vi "test1-SystemLevelModuleInListModuleAPI.vi"(8 "error in (no error)":errorcluster, 11 "TestCase in":refnum<class "testcase-CSMSystemLevelModule.lvclass">) -> (0 "error out":errorcluster, 3 "TestCase out":refnum<class "testcase-CSMSystemLevelModule.lvclass">)   [LabVIEW 2017, in "testcase-CSMSystemLevelModule.lvclass"]
uses:
  testcase-CSMSystemLevelModule.lvclass
  src/user.lib/_NEVSTOP/Communicable State Machine(CSM)/_Support/Typedef/_CSM_List Module Scope.ctl
  <vilib>/addons/_JKI Toolkits/VI Tester/TestCase.llb/TestCase.lvclass
  src/user.lib/_NEVSTOP/Communicable State Machine(CSM)/Communicable State Machine.lvlib
  C:/Program Files (x86)/National Instruments/LabVIEW 2017/vi.lib/addons/_JKI Toolkits/VI Tester/TestCase.llb/TestCase.lvclass
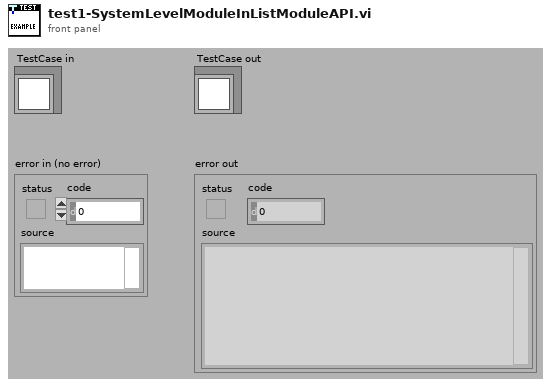
[diagram p1: front panel]
types:
  T1 = typedef "Communicable State Machine.lvlib/_CSM_List Module Scope.ctl" = enum16{"Normal", "System Only", "All"}
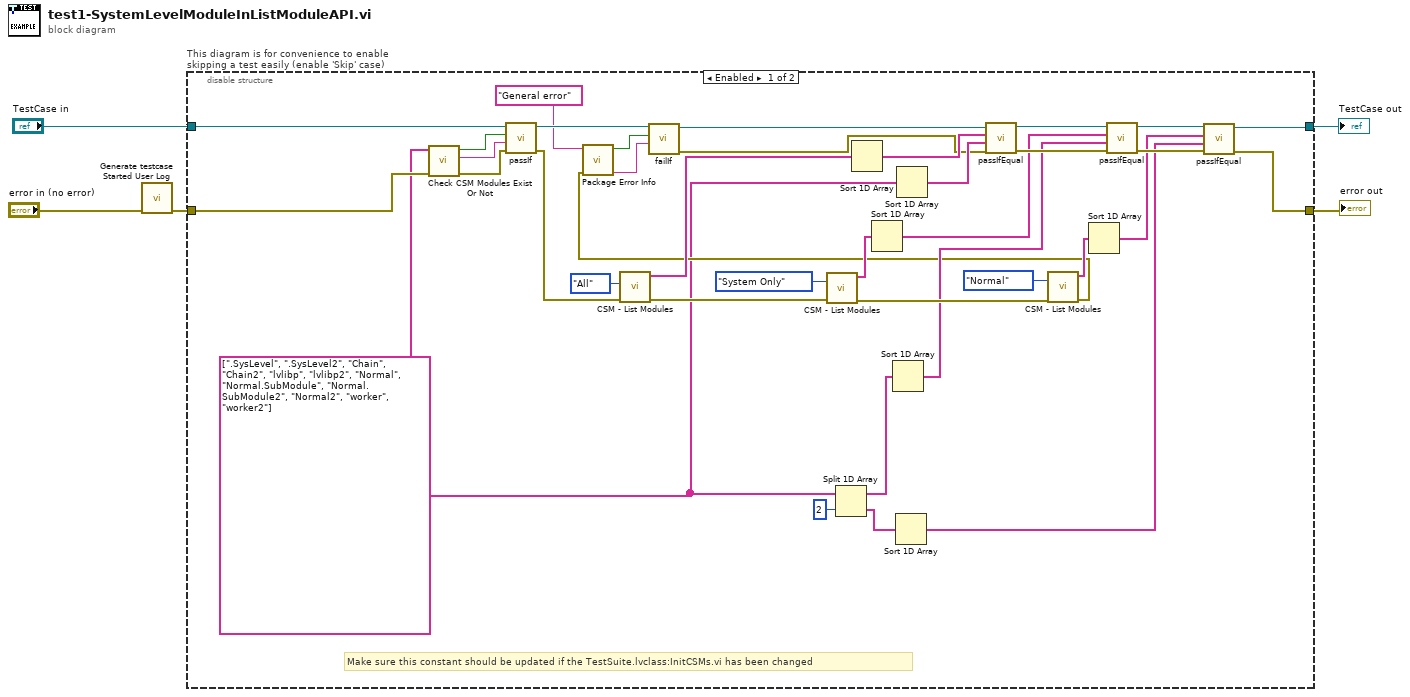
[diagram p0: block diagram]
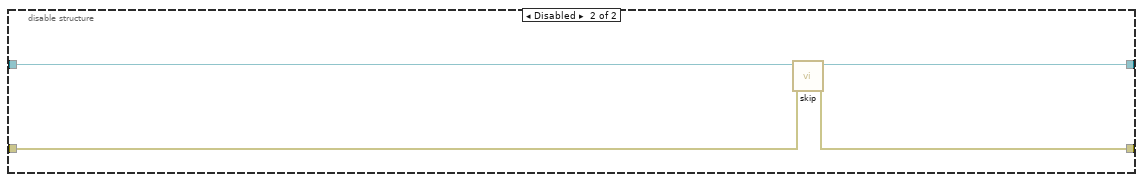
[diagram p2: hidden frame]
diagram:
  n1 = call "Generate testcase Started User Log.vi"("Error In"="error in (no error)") -> ("error out"=w1:errorcluster)  [unwired: 10 in]
  n2 = disable-structure "This diagram is for convenience to enable skipping a test easily (enable 'Skip' case)" shown="Enabled" {
    disable-tunnel: "TestCase in" -> [w16 w46]
    disable-tunnel: [w32 w44] -> w2
    disable-tunnel: [w29 w45] -> w4
    disable-tunnel: w1 -> [w15 w43]
    frame Enabled {
      w6 = string[] [".SysLevel", ".SysLevel2", "Chain", "Chain2", "lvlibp", "lvlibp2", "Normal", "Normal.SubModule", "Normal.SubModule2", "Normal2", "worker", "worker2"] ("Module Names in All Scope")
      # "Make sure this constant should be updated if the TestSuite.lvclass:InitCSMs.vi has been changed"
      n3 = call "Check CSM Modules Exist Or Not.vi"("error in"=w15, "CSM names in"=w6) -> ("error out"=w17:errorcluster, "Debug string"=w18:string, "All Modules Exist?"=w19:bool)  [unwired: 7 in]
      n4 = call-dynamic "passIf.vi"("error in (no error)"=w17, "message (\"\")"=w18, "pass"=w19, "TestCase in"=w16) -> ("error out"=w14:errorcluster, "TestCase out"=w11:refnum<class "testcase-CSMSystemLevelModule.lvclass">)  [unwired: 6 in]
      n5 = call "CSM - List Modules.vi"("Error In"=w14, "Scope (Normal)"=_CSM_List_Module_Scope."All") -> ("error out"=w39:errorcluster, "Module Names"=w37:string[])  [unwired: 8 in]
      n6 = call "CSM - List Modules.vi"("Error In"=w39, "Scope (Normal)"=_CSM_List_Module_Scope."System Only") -> ("error out"=w38:errorcluster, "Module Names"=w28:string[])  [unwired: 8 in]
      n7 = Split 1D Array(array=w6, index=2) -> (first subarray=w24:string[], second subarray=w23:string[])
      n8 = Sort 1D Array(array=w37) -> (sorted array=w36:string[])
      n9 = Sort 1D Array(array=w28) -> (sorted array=w27:string[])
      n10 = Sort 1D Array(array=w24) -> (sorted array=w26:string[])
      n11 = Sort 1D Array(array=w23) -> (sorted array=w20:string[])
      n12 = Sort 1D Array(array=w6) -> (sorted array=w35:string[])
      n13 = call "CSM - List Modules.vi"("Error In"=w38, "Scope (Normal)"=_CSM_List_Module_Scope."Normal") -> ("error out"=w9:errorcluster, "Module Names"=w22:string[])  [unwired: 8 in]
      n14 = call "Package Error Info.vi"("error in"=w9, "String in"="General error") -> ("packed error info out"=w12:string, "error status"=w13:bool)  [unwired: 8 in]
      n15 = call-dynamic "failIf.vi"("message (\"\")"=w12, "fail"=w13, "TestCase in"=w11) -> ("error out"=w7:errorcluster, "TestCase out"=w10:refnum<class "testcase-CSMSystemLevelModule.lvclass">)  [unwired: 7 in]
      n16 = call-dynamic "passIfEqual.vi"("error in (no error)"=w7, "y"=w35, "x"=w36, "TestCase in"=w10) -> ("error out"=w31:errorcluster, "TestCase out"=w34:refnum<class "testcase-CSMSystemLevelModule.lvclass">)  [unwired: 6 in]
      n17 = Sort 1D Array(array=w22) -> (sorted array=w21:string[])
      n18 = call-dynamic "passIfEqual.vi"("error in (no error)"=w31, "y"=w26, "x"=w27, "TestCase in"=w34) -> ("error out"=w30:errorcluster, "TestCase out"=w33:refnum<class "testcase-CSMSystemLevelModule.lvclass">)  [unwired: 6 in]
      n19 = call-dynamic "passIfEqual.vi"("error in (no error)"=w30, "y"=w20, "x"=w21, "TestCase in"=w33) -> ("error out"=w29:errorcluster, "TestCase out"=w32:refnum<class "testcase-CSMSystemLevelModule.lvclass">)  [unwired: 6 in]
    }
    frame Disabled {
      # "skip test result while test is under development"
      n20 = call <vilib>:"skip.vi"("error in (no error)"=w43, "TestCase in"=w46) -> ("error out"=w45:errorcluster, "TestCase out"=w44:refnum<class "testcase-CSMSystemLevelModule.lvclass">)  [unwired: 8 in]
    }
  }
  "error out" <- w4
  "TestCase out" <- w2
